vi "Set Dict.vi"(10 "Dict":map{string, map{string, string}}(c390), 11 "Object Dictionary in":refnum<class "Object Dictionary.lvclass">) -> (3 "Object Dictionary out":refnum<class "Object Dictionary.lvclass">)   [LabVIEW 2024, in "Object Dictionary.lvclass"]
uses:
  Object Dictionary.lvclass
  Object Dictionary.lvclass/Object Dictionary.ctl
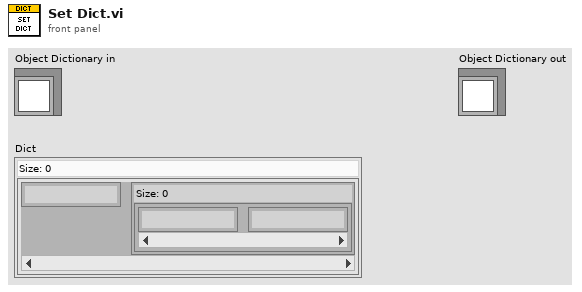
[diagram p1: front panel]
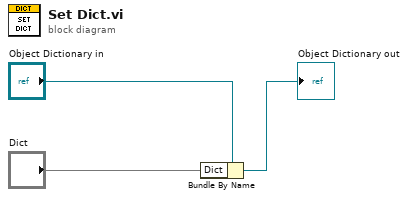
[diagram p0: block diagram]
diagram:
  n1 = Bundle By Name(cluster="Object Dictionary in", "Dict"="Dict") -> (→"Object Dictionary out":refnum<class "Object Dictionary.lvclass">)
